vi "GetType.vi"(8 "error in (no error)":errorcluster, 11 "Configure StopVelocity Msg":refnum<class "Configure StopVelocity Msg.lvclass">) -> (0 "error out":errorcluster, 2 "Data Sample":variant, 3 "Configure StopVelocity Msg":refnum<class "Configure StopVelocity Msg.lvclass">)   [LabVIEW 2015, in "CS++Motor.lvlib" / "Configure StopVelocity Msg.lvclass"]
uses:
  Configure StopVelocity Msg.lvclass
  Configure StopVelocity Msg.lvclass/Configure StopVelocity Msg.ctl
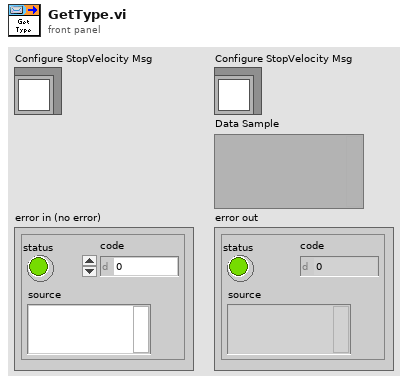
[diagram p1: front panel]
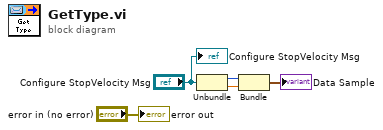
[diagram p0: block diagram]
diagram:
  n1 = Unbundle("Configure StopVelocity Msg") -> (w2:u8, w1:dbl)
  n2 = Bundle("AxisNumber"=w2, "StopVelocity"=w1) -> (→"Data Sample":cluster{"AxisNumber":u8, "StopVelocity":dbl})  [unwired: 1 in]
  "error out" <- "error in (no error)"
  "Configure StopVelocity Msg" <- "Configure StopVelocity Msg"
